vi "sinnn.vi"() -> ()   [LabVIEW 2015]
uses:
  <vilib>/Analysis/NI_AALBase.lvlib
panel:
  in  "End":dbl
  in  "Start":dbl
  out "dx/dy End 3":dbl
  out "dx/dy Start 3":dbl
  out "x < y?":bool
  out "x/y":dbl
  out "dx/dy End 2":dbl
  out "dx/dy Start 2":dbl
  out "Sin Connection":dbl[](graph)
  in  "dx/dy End":dbl
  in  "dx/dy Start":dbl
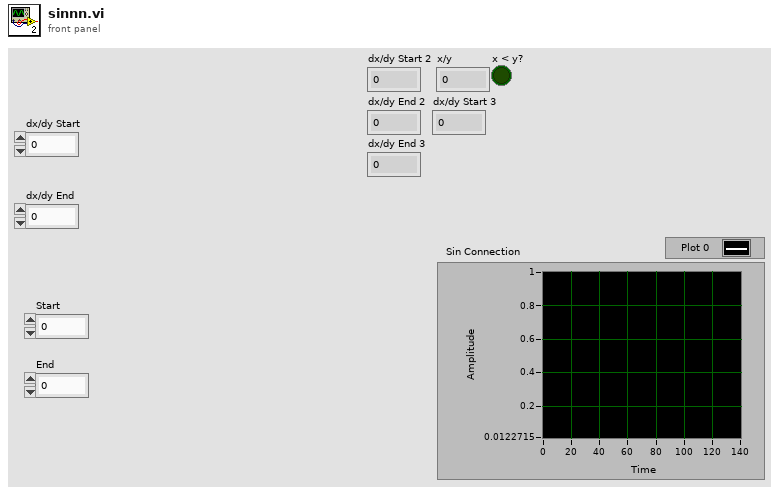
[diagram p1: front panel]
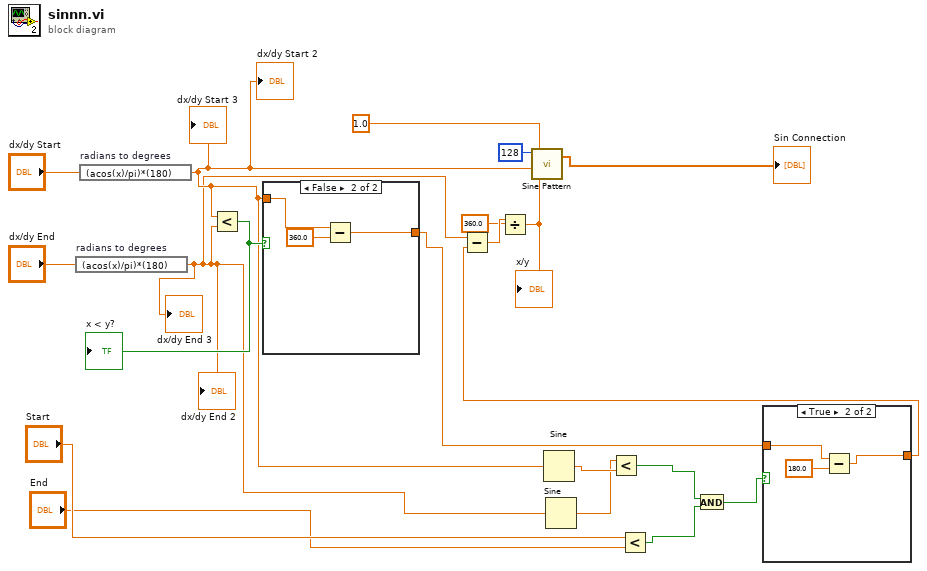
[diagram p0: block diagram]
diagram:
  n1 = expression code="(acos(x)/pi)*(180)" "radians to degrees"("dx/dy End") -> (w10:dbl)
  "dx/dy End 2" <- w10
  "dx/dy End 3" <- w10
  n2 = expression code="(acos(x)/pi)*(180)" "radians to degrees"("dx/dy Start") -> (w11:dbl)
  "dx/dy Start 2" <- w11
  "dx/dy Start 3" <- w11
  n3 = Less?(x=w11, y=w10) -> (x < y?=w15:bool)
  "x < y?" <- w15
  n4 = case shown="False" w15 {
    tunnel: w11 -> [w21 w24]
    tunnel: [w21 w22] -> w8
    frame True {
    }
    frame False {
      n5 = Subtract(x=w24, y=360.0) -> (x-y=w22:dbl)
    }
  }
  n6 = Sine(x=w11) -> (sin(x)=w4:dbl)
  n7 = Sine(x=w10) -> (sin(x)=w3:dbl)
  n8 = Less?(x=w3, y=w4) -> (x < y?=w5:bool)
  n9 = Less?(x="Start", y="End") -> (x < y?=w6:bool)
  n10 = And(x=w5, y=w6) -> (x .and. y?=w9:bool)
  n11 = case shown="True" w9 {
    tunnel: w8 -> [w25 w28]
    tunnel: [w25 w26] -> w7
    frame False {
    }
    frame True {
      n12 = Subtract(x=w28, y=180.0) -> (x-y=w26:dbl)
    }
  }
  n13 = Subtract(x=w10, y=w7) -> (x-y=w14:dbl)
  n14 = Divide(x=w14, y=360.0) -> (x/y=w12:dbl)
  "x/y" <- w12
  n15 = call <vilib>:"Sine Pattern.vi"("cycles"=w12, "phase(degrees)"=w11, "amplitude"=1.0, "samples"=128) -> ("Sinusoidal Pattern"=→"Sin Connection":dbl[])  [unwired: 1 out]
